vi "rx0.vi"(1 "Cluster 2":T1) -> (0 "Cluster":T1)   [LabVIEW 2010]
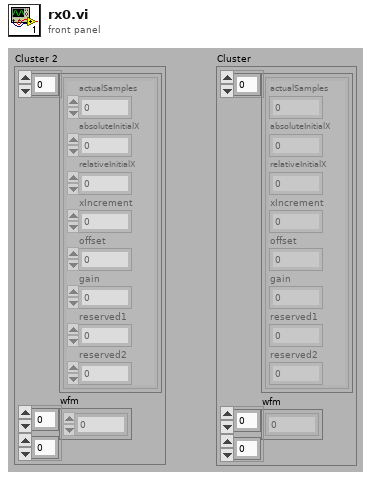
[diagram p1: front panel]
types:
  T1 = cluster{cluster{"actualSamples":i32, "absoluteInitialX":dbl, "relativeInitialX":dbl, "xIncrement":dbl, "offset":dbl, "gain":dbl, "reserved1":dbl, "reserved2":dbl}[], "wfm":i16[][]}
  T2 = cluster{"actualSamples":i32, "absoluteInitialX":dbl, "relativeInitialX":dbl, "xIncrement":dbl, "offset":dbl, "gain":dbl, "reserved1":dbl, "reserved2":dbl}[]
  T3 = cluster{"actualSamples":i32, "absoluteInitialX":dbl, "relativeInitialX":dbl, "xIncrement":dbl, "offset":dbl, "gain":dbl, "reserved1":dbl, "reserved2":dbl}
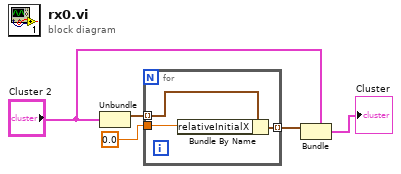
[diagram p0: block diagram]
diagram:
  n1 = Unbundle("Cluster 2") -> (w2:T2)  [unwired: 1 out]
  n2 = for {
    tunnel: w2 -> [w8] mode=indexing
    tunnel: [w7] -> w4 mode=indexing
    tunnel: 0.0 ("relativeInitialX") -> [w6]
    n3 = Bundle By Name(cluster=w8, "relativeInitialX"=w6) -> (w7:T3)
  }
  n4 = Bundle(cluster="Cluster 2", w4) -> (→"Cluster":T1)  [unwired: 1 in]
